vi "Create Report.vi"(10 "error in (no error)":errorcluster, 11 "Execution":T2) -> (2 "error out":errorcluster, 3 "Report":T1)   [LabVIEW 2020, in "TSS.lvlib" / "Engine.lvclass"]
uses:
  Engine.lvclass
  Execution/Typedefs/Session Handle.ctl
  Execution/Execution.lvclass
  Report/Typedefs/Session Handle.ctl
  Report/Report.lvclass
  Execution/Get Execution Ref.vi
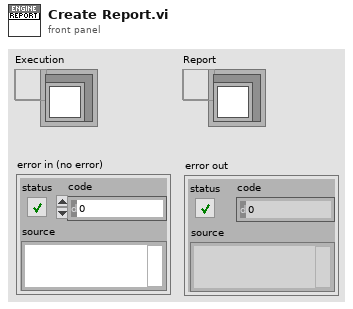
[diagram p1: front panel]
types:
  T1 = typedef "TSS.lvlib/Report.lvclass/Session Handle.ctl" = refnum<data-value>
  T2 = typedef "TSS.lvlib/Execution.lvclass/Session Handle.ctl" = refnum<data-value>
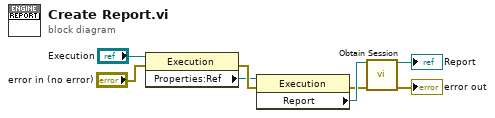
[diagram p0: block diagram]
diagram:
  n1 = property class="Execution"(reference="Execution", error in="error in (no error)") -> (error out=w8:errorcluster, "Properties:Ref"=w7:refnum<k7>)  [unwired: 1 out]
  n2 = property class="Execution"(reference=w7, error in=w8) -> (error out=w3:errorcluster, "Report"=w4:refnum<k7>)  [unwired: 1 out]
  n3 = call "Obtain Session.vi"("Report"=w4, "error in (no error)"=w3) -> ("Session Handle"=→"Report":T1, "error out"=→"error out":errorcluster)  [unwired: 12 in]
